vi "Initialize.vi"() -> ()   [LabVIEW 2017, in "LabPack.lvlib"]
uses:
  LabPack.lvlib
panel:
  out "Shared Library Out":path
  out "Error Out":errorcluster
  in  "Error In":errorcluster
  in  "Shared Library In":path
  in  "Unload":bool
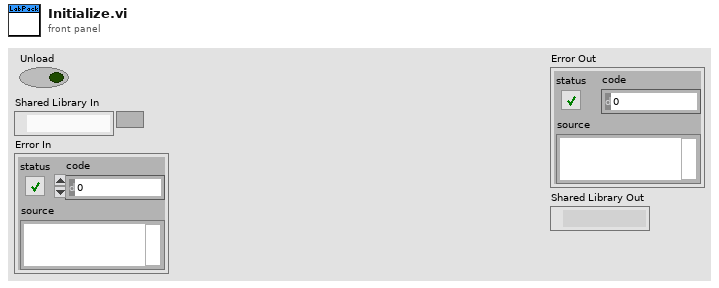
[diagram p1: front panel]
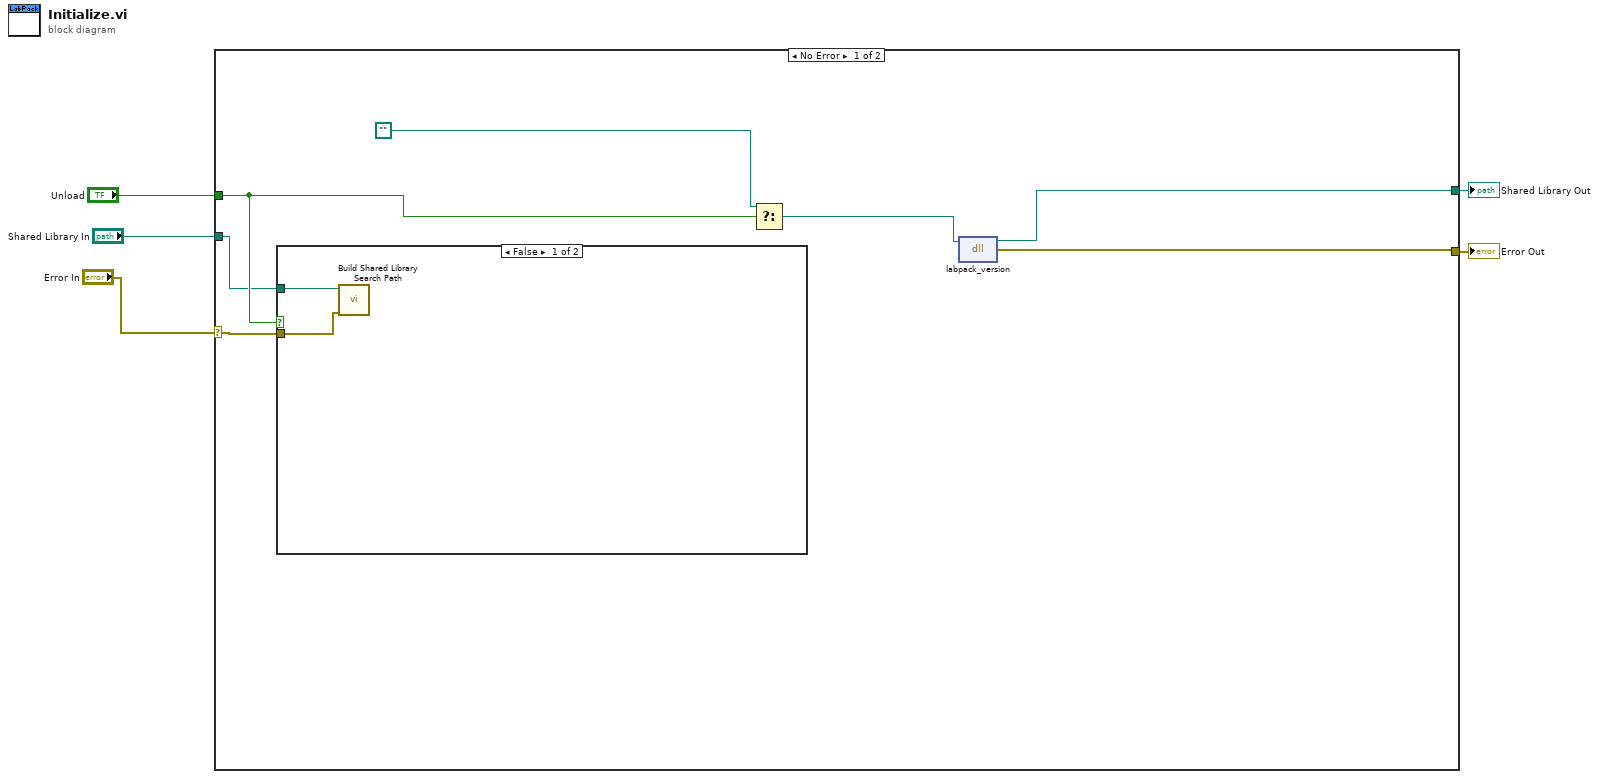
[diagram p0: block diagram]
diagram:
  n1 = case shown="No Error" "Error In" {
    selector: "Error In" -> [w6 _]
    tunnel: "Unload" -> [w8 _]
    tunnel: "Shared Library In" -> [w7 _]
    tunnel: [w10 _] -> w2
    tunnel: [w9 _] -> w1
    frame No Error {
      n2 = case shown="False" w8 {
        tunnel: w7 -> [w14 _]
        tunnel: w6 -> [w13 _]
        frame False {
          n3 = call "Build Shared Library Search Path.vi"("Error In"=w13, "LabPack Shared Library"=w14) -> ()  [unwired: 8 in, 2 out]
        }
        frame True {
        }
      }
      n4 = Select(t=path "", s=w8) -> (s? t:f=w11:path)  [unwired: 1 in]
      n5 = dll-call lib="D:/Users/cfield/Code/MessagePack/LabPack/LabVIEW/trunk/src/LabPack/Private/labpack-x64.dll" fn="labpack_version"(path in=w11) -> (path out=w9:path, error out=w10:errorcluster)  [unwired: 3 in]
    }
    frame Error {
    }
  }
  "Error Out" <- w2
  "Shared Library Out" <- w1
